vi "setForceAboutDirection.vi"(11 "kconstant":dbl) -> (3 "DesiredFM":dbl[](array[numeric]))   [LabVIEW 2017]
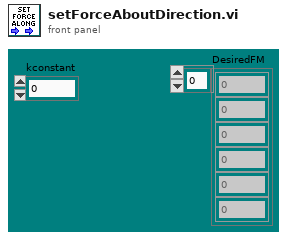
[diagram p1: front panel]
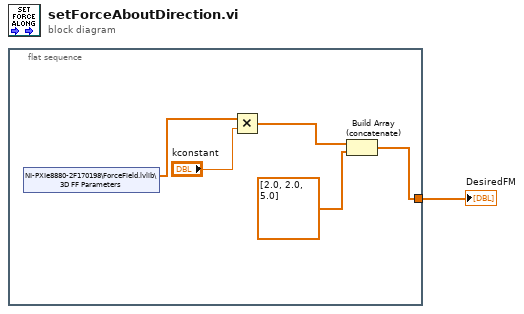
[diagram p0: block diagram]
diagram:
  n1 = flat-sequence {
    tunnel: [w3] -> w1
    frame #0 {
      n2 = shared-variable "NI-PXIe8880-2F170198\\ForceField.lvlib\\3D FF Parameters"() -> (w6:dbl[])  [unwired: 1 in, 1 out]
      n3 = Multiply(x=w6, y="kconstant") -> (x*y=w4:dbl[])
      n4 = Build Array (concatenate)(w4, dbl[] [2.0, 2.0, 5.0] ("array")) -> (w3:dbl[])
    }
  }
  "DesiredFM" <- w1
